vi "序列号写入.vi"(11 "序列号:":string) -> (2 "确认 2":bool, 3 "序列号输出":string)   [LabVIEW 2016, in "斯坦道CODMn.lvlib"]
panel:
  in  "取消":bool
  in  "确认":bool
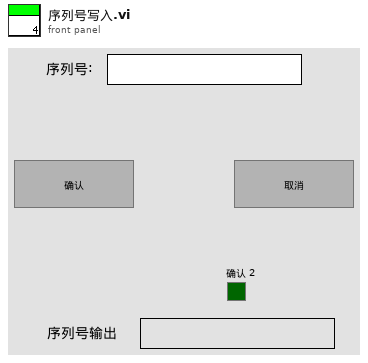
[diagram p1: front panel]
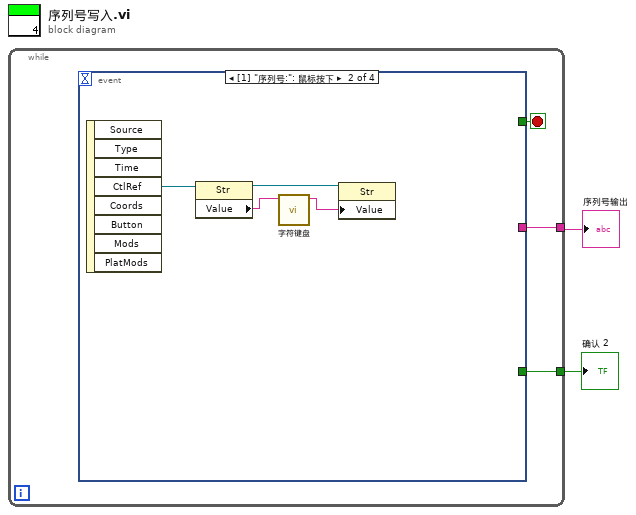
[diagram p0: block diagram]
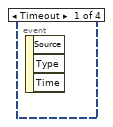
[diagram p2: hidden frame]
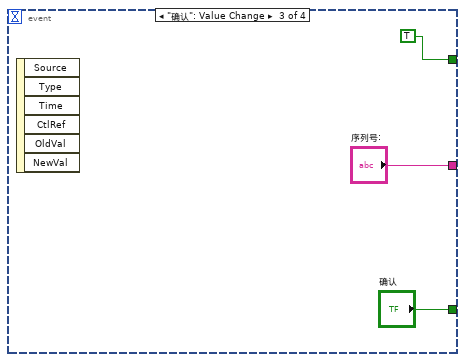
[diagram p3: hidden frame]
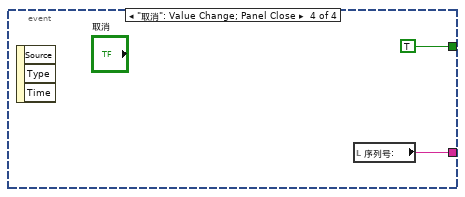
[diagram p4: hidden frame]
diagram:
  n1 = while {
    tunnel: [w5] -> w1
    tunnel: [w3] -> w2
    stop <- w4 stop-if-true
    n2 = event shown="[1] \"序列号:\": 鼠标按下" {
      selector: _ -> [_ _ _ _]
      dyn-events: _ -> [_ _ _ _]
      timeout: _ -> [_ _ _ _]
      tunnel: [_ _ "序列号:" w13] -> w5
      tunnel: [_ _ TRUE TRUE] -> w4
      tunnel: [_ _ "确认" _] -> w3
      event Timeout {
        n3 = event-data() -> ()  [unwired: 1 in, 3 out]
      }
      event "序列号:": Mouse Down {
        n4 = event-data() -> ("CtlRef"=w9:refnum<vi>)  [unwired: 1 in, 7 out]
        n5 = property class="Str"(reference=w9) -> (reference out=w8:refnum<vi>, "Value"=w7:string)  [unwired: 1 in, 1 out]
        n6 = call "字符键盘.vi"("原值"=w7) -> ("x+y"=w6:string)  [unwired: 10 in]
        n7 = property class="Str"(reference=w8, "Value"=w6) -> ()  [unwired: 1 in, 2 out]
      }
      event "确认": Value Change {
        n8 = event-data() -> ()  [unwired: 1 in, 6 out]
      }
      event "取消": Value Change; Panel Close {
        n9 = event-data() -> ()  [unwired: 1 in, 3 out]
        n10 = local read "序列号:"() -> (w13:string)
      }
    }
  }
  "确认 2" <- w2
  "序列号输出" <- w1
